vi "MindwavePrecise.vi"(3 "error in (no error) input":errorcluster, 4 "Control Box":u16(ring) items=["GetRAWEEG", "GetBigPacket", "GetStream"], 5 "VISA resource name input":refnum<visa-resource-name>) -> (0 "error out":errorcluster, 1 "MindWave":T1, 2 "VISA resource name out":refnum<visa-resource-name>)   [LabVIEW 2011, in "Neurosky.lvlib"]
uses:
  Users/Isaias/Documents/GitHub/Neurosky/Neurosky.lvlib
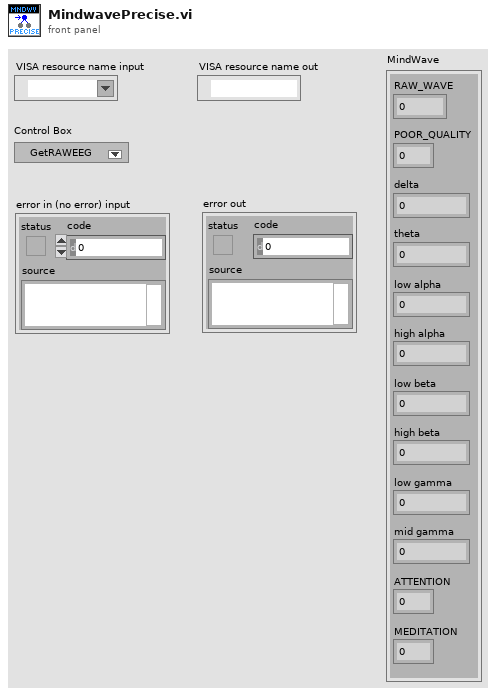
[diagram p1: front panel]
types:
  T1 = cluster{"RAW_WAVE":i16, "POOR_QUALITY":u8, "delta":sgl, "theta":sgl, "low alpha":sgl, "high alpha":sgl, "low beta":sgl, "high beta":sgl, "low gamma":sgl, "mid gamma":sgl, "ATTENTION":u8, "MEDITATION":u8}
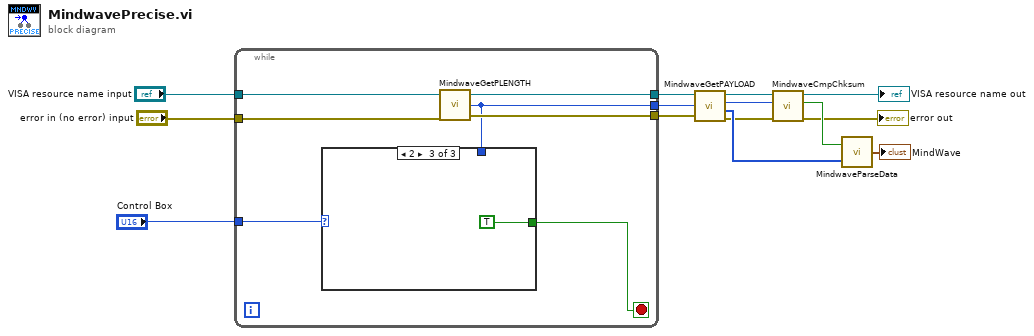
[diagram p0: block diagram]
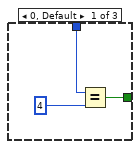
[diagram p2: hidden frame]
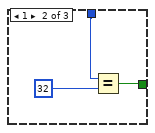
[diagram p3: hidden frame]
diagram:
  n1 = while {
    tunnel: "Control Box" -> [w21]
    tunnel: [w20] -> w4
    tunnel: [w19] -> w6
    tunnel: [w16] -> w5
    tunnel: "error in (no error) input" -> [w18]
    tunnel: "VISA resource name input" -> [w17]
    stop <- w15 stop-if-true
    n2 = call <userlib>:"MindwaveGetPLENGTH.vi"("error in (no error) input"=w18, "VISA resource name input"=w17) -> ("error out"=w19:errorcluster, "[PLENGTH]"=w16:u8, "VISA resource name out"=w20:refnum<visa-resource-name>)  [unwired: 1 in]
    n3 = case shown="2" w21 {
      tunnel: w16 -> [w23 w25 _]
      tunnel: [w22 w26 TRUE] -> w15
      frame 0, Default {
        n4 = Equal?(x=w23, y=4) -> (x = y?=w22:bool)
      }
      frame 1 {
        n5 = Equal?(x=w25, y=32) -> (x = y?=w26:bool)
      }
      frame 2 {
      }
    }
  }
  n6 = call <userlib>:"MindwaveGetPAYLOAD.vi"("error input"=w6, "[PLENGTH]"=w5, "VISA resource name input"=w4) -> ("error out"=w7:errorcluster, "[PAYLOAD]"=w8:u8[], "[CHECKSUM]"=w10:u8, "VISA resource name out"=w11:refnum<visa-resource-name>)  [unwired: 1 in]
  n7 = call <userlib>:"MindwaveCmpChksum.vi"("error in (no error) input"=w7, "[CHECKSUM] - CALCULATED"=w10, "VISA resource name input"=w11) -> ("error out"=→"error out":errorcluster, "canParseData?"=w9:bool, "VISA resource name out"=→"VISA resource name out":refnum<visa-resource-name>)  [unwired: 2 in]
  n8 = call <userlib>:"MindwaveParseData.vi"("RAW_ARRAY"=w8, "canParseData?"=w9) -> ("MindWave"=→"MindWave":T1)
